vi "Write time series variant.vi"(0 "InfluxDB in":refnum<class "InfluxDB Client.lvclass">, 5 "Database name":string, 7 "Series name":string, 9 "Precision (ms)":T1=enum."milliseconds", 11 "error in (no error)":errorcluster, 12 "Variant data":variant) -> (4 "InfluxDB out":refnum<class "InfluxDB Client.lvclass">, 15 "error out":errorcluster)   [LabVIEW 2013, in "InfluxDB Client.lvclass"]
doc: "Writes time series data (Variant format) to a specific database."
uses:
  InfluxDB Client.lvclass
  Time precision.ctl
  InfluxDB Client.lvclass/InfluxDB Client.ctl
  <vilib>/httpClient/POSTBuffer.vi
  <vilib>/httpClient/LabVIEWHTTPClient.lvlib
panel:
  out "Status":string
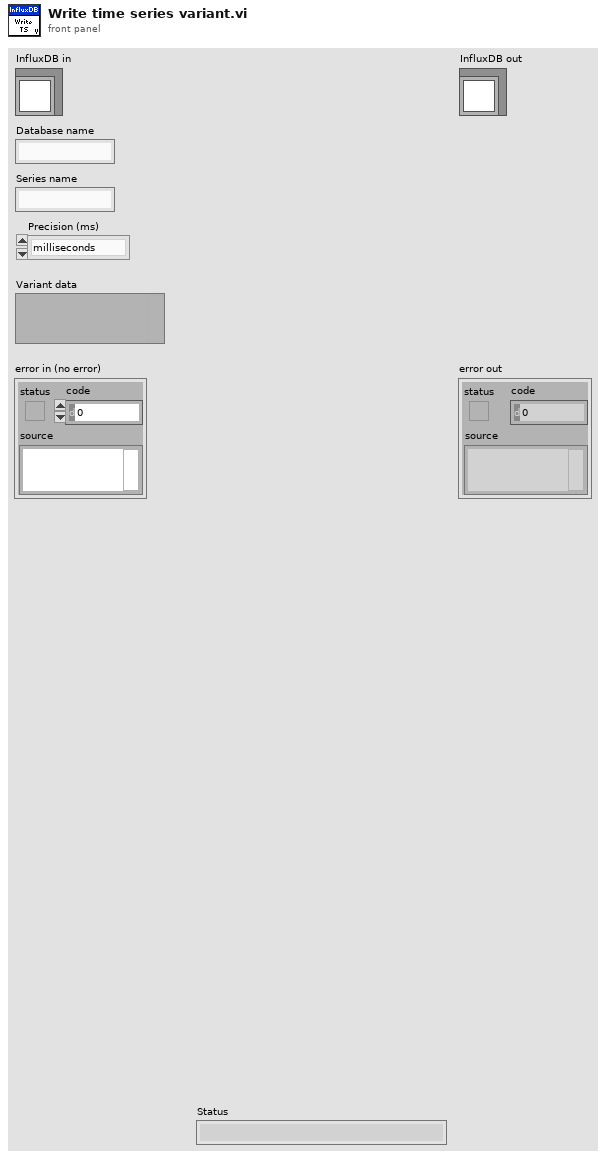
[diagram p1: front panel]
types:
  T1 = typedef "InfluxDB Client.lvclass/Time precision.ctl" = enum16{"seconds", "milliseconds", "microseconds"}
  T2 = typedef "LabVIEWHTTPClient.lvlib/ClientHandle.ctl" = refnum<k1>
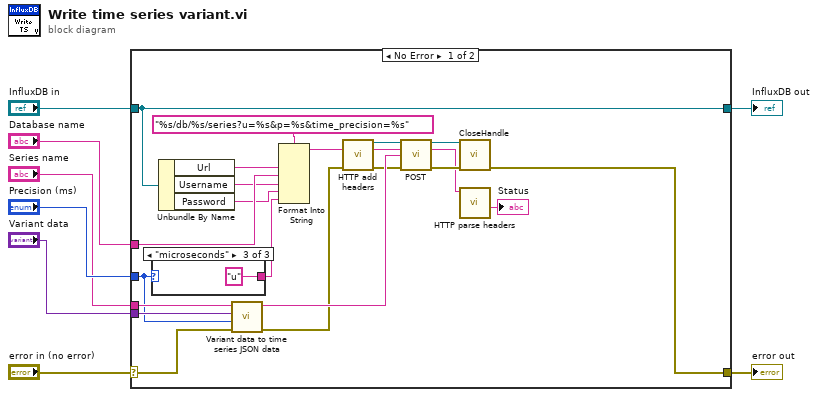
[diagram p0: block diagram]
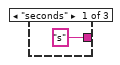
[diagram p2: hidden frame]
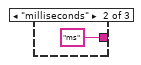
[diagram p3: hidden frame]
diagram:
  n1 = case shown="No Error" "error in (no error)" {
    selector: "error in (no error)" -> [w14 w34]
    tunnel: [w23 w34] -> w7
    tunnel: [w29 w33] -> w5
    tunnel: "InfluxDB in" -> [w29 w33]
    tunnel: "Database name" -> [w20 _]
    tunnel: "Precision (ms)" -> [w9 _]
    tunnel: "Variant data" -> [w17 _]
    tunnel: "Series name" -> [w15 _]
    frame No Error {
      n2 = case shown="\"microseconds\"" w9 {
        tunnel: ["s" ("Database name") "ms" ("Database name") "u" ("Database name")] -> w10
        frame "seconds" {
        }
        frame "milliseconds" {
        }
        frame "microseconds" {
        }
      }
      n3 = Unbundle By Name(w29) -> ("Url"=w27:string, "Username"=w19:string, "Password"=w18:string)
      n4 = call "Variant data to time series JSON data.vi"("error in (no error)"=w14, "Precision (ms)"=w9, "Data"=w17, "Series name"=w15) -> ("error out"=w13:errorcluster, "JSON data"=w16:string)  [unwired: 6 in]
      n5 = Format Into String(format string="%s/db/%s/series?u=%s&p=%s&time_precision=%s" ("url"), w27, w20, w19, w18, w10) -> (resulting string=w24:string)  [unwired: 2 in, 1 out]
      n6 = call "HTTP add headers.vi"("error in (no error)"=w13) -> ("client handle out"=w11:T2, "error out"=w12:errorcluster)  [unwired: 13 in]
      n7 = call-poly <vilib>:"POST.vi"("client handle"=w11, "url"=w24, "buffer"=w16, "error in (no error)"=w12) -> ("client handle out"=w26:T2, "headers"=w22:string, "error out"=w25:errorcluster)  [unwired: 8 in, 1 out]
      n8 = call <vilib>:"CloseHandle.vi"("client handle"=w26, "error in (no error)"=w25) -> ("error out"=w23:errorcluster)  [unwired: 13 in]
      n9 = call "HTTP parse headers.vi"("HTTP headers"=w22) -> ("Status"=→"Status":string)  [unwired: 8 in, 2 out]
    }
    frame Error {
    }
  }
  "error out" <- w7
  "InfluxDB out" <- w5
